vi "Optical Intrinsic Imaging with Optogenetic Stimulation_LED_3.0_w_Neuro.vi"() -> ()   [LabVIEW 2015]
uses:
  <vilib>/userdefined/High Color/IMAQdx.ctl
  <vilib>/vision/driver/IMAQdx.llb/IMAQdx Camera Control Mode.ctl
  <vilib>/DAQmx/write.llb/DAQmx Write (Analog 1D DBL 1Chan NSamp).vi
  <vilib>/DAQmx/read.llb/DAQmx Read (Analog 1D Wfm NChan NSamp).vi
  <vilib>/DAQmx/write.llb/DAQmx Write (Digital 1D Bool 1Chan 1Samp).vi
  <vilib>/DAQmx/create/channels.llb/DAQmx Create Channel (CO-Pulse Generation-Frequency).vi
  <vilib>/DAQmx/configure/timing.llb/DAQmx Timing (Implicit).vi
  <vilib>/DAQmx/create/channels.llb/DAQmx Create Channel (DO-Digital Output).vi
  <vilib>/DAQmx/create/channels.llb/DAQmx Create Channel (AI-Voltage-Basic).vi
  <vilib>/DAQmx/configure/timing.llb/DAQmx Timing (Sample Clock).vi
  <vilib>/DAQmx/configure/trigger.llb/DAQmx Start Trigger (Digital Edge).vi
  <vilib>/Waveform/DWDTOps.llb/DWDT Digital to Boolean Array.vi
  <vilib>/DAQmx/create/channels.llb/DAQmx Create Channel (AO-Voltage-Basic).vi
  <vilib>/DAQmx/miscellaneous.llb/DAQmx Fill In Error Info.vi
  <vilib>/vision/driver/NI_Vision_Acquisition_Software.lvlib
  <resource>/objmgr/daqmx.rc
panel:
  out "LED":bool
  out "Ball Velocity":waveform(dbl)(graph)={"t0"=timestamp(3636461995.1352177 s since 1904-01-01), "dt"=4.999999999999997e-05, "Y"=[-0.0010089086442716115, -0.001653132464493098, -0.0008478526887906051, -0.0008478526887906051, -0.001492076509693054, -0.001492076509693054, -0.0011699645995823372, -0.0008478526887906051, -0.0011699645995823372, -0.001492076509693054, -0.0013310205547228094], "attributes"=variant("NI_ChannelName"=variant(string "Dev1/ai0"), "NI_UnitDescription"=variant(string "Volts"))}
  out "Right Pad":bool
  out "Control":bool
  out "Left Pad":bool
  in  "Sol Stim Parameters":cluster{"Fs":dbl, "Samples":dbl}
  in  "LED Stim Parameters":cluster{"Fs":dbl, "Samples":dbl}
  in  "Sol Duty Cycle (%)":dbl=50.0
  in  "Sol Frequency":dbl=1.0
  in  "Sol Stim Duration (s)":dbl=1.0
  in  "LED duty cycle (%)":dbl=10.0
  in  "LED Frequency":dbl=10.0
  in  "LED Stim Duration (s)":dbl=2.0
  out "Stimulus Presentation Order":digitalwaveform[](graph)=[{"t0"=timestamp(0 s since 1904-01-01), "dt"=5e-05, "Y"={"transitions"=[], "data"=array6000000x1[6000000 elements]}}, {"t0"=timestamp(0 s since 1904-01-01), "dt"=5e-05, "Y"={"transitions"=[], "data"=array6000000x1[6000000 elements]}}, {"t0"=timestamp(0 s since 1904-01-01), "dt"=5e-05, "Y"={"transitions"=[], "data"=array6000000x1[6000000 elements]}}, {"t0"=timestamp(0 s since 1904-01-01), "dt"=5e-05, "Y"={"transitions"=[], "data"=array6000000x1[6000000 elements]}}]
  out "Solenoid Stim":digitalwaveform(graph)={"t0"=timestamp(0 s since 1904-01-01), "dt"=5e-05, "Y"={"transitions"=[], "data"=array20000x1[20000 elements]}}
  out "Dalsa Image":T1(plugin-control)
  in  "Trigger Solenoids":bool
  in  "WebCam\nFrame Rate":u32=15
  in  "Session Notes:":string[](array[string])=["QZ", "QZ_CHR01", "RH", "10", "0", "1", "n"]
  in  "Ai7":string="LED"
  in  "Ai6":string="MUA"
  in  "Ai5":string="LFP"
  in  "Ai4":string="Neuro\nSol"
  in  "Ai3":string="Right \nPad"
  in  "Ai2":string="Ctrl\nPad"
  in  "Ai1":string="Left Pad"
  in  "Ai0":string="VBall"
  in  "Flash LED":bool=TRUE
  in  "Trial Offset (s)":dbl=10.0
  in  "Time Between Stims (s)":dbl=30.0
  in  "Right Pad":dbl
  in  "Left Pad":dbl
  in  "Control":dbl
  in  "LED":dbl=5.0
  in  "Target Path":path=path "E:/Qingguang" caption="Final Saved Location for Files"
  in  "Analog Sampling Rate":dbl=20000.0 format="%0.0f"
  out "Analog file name":string="190326_12_18_1026"
  in  "physical channels":tag="Dev1/ai0:7"
  out "Actual WebCam Frame Rate":dbl(knob) scale=0.0..30.0
  out "WebCam":T1(plugin-control)
  out "Finished Acquiring":bool
  out "Trial Time Elapsed (Min)":cluster{dbl, dbl}(slide)={5.0, 1.6085833333333333} scale=0.0..5.0
  in  "Recording Time (min)":dbl=5.0 min=0.5 max=10.0 step=0.5
  in  "Temp Path":path=path "C:/LabView Direct Files" caption="Temporary Path for Streamed Data"
  in  "Dalsa\nFrame Rate":dbl=30.0
  out "Last Dalsa Buffer":i32=284
  in  "Stop":bool
  out "Actual Dalsa Frame Rate":dbl(knob) scale=0.0..60.0
  # "Experimenter"
  # "Animal ID"
  # "Imaged Hemisphere (RH/LH)"
  # "Solenoid Pressure (psi)"
  # "Isoflurane Time (military)"
  # "Session Number"
  # "Flash LEDs? (y/n)"
  # "Setup Stimulation:"
  # "File Settings:"
  # "Analog Acquisition Setup:"
  # "Camera Acquisition Setup:"
  # "BNC Pinout"
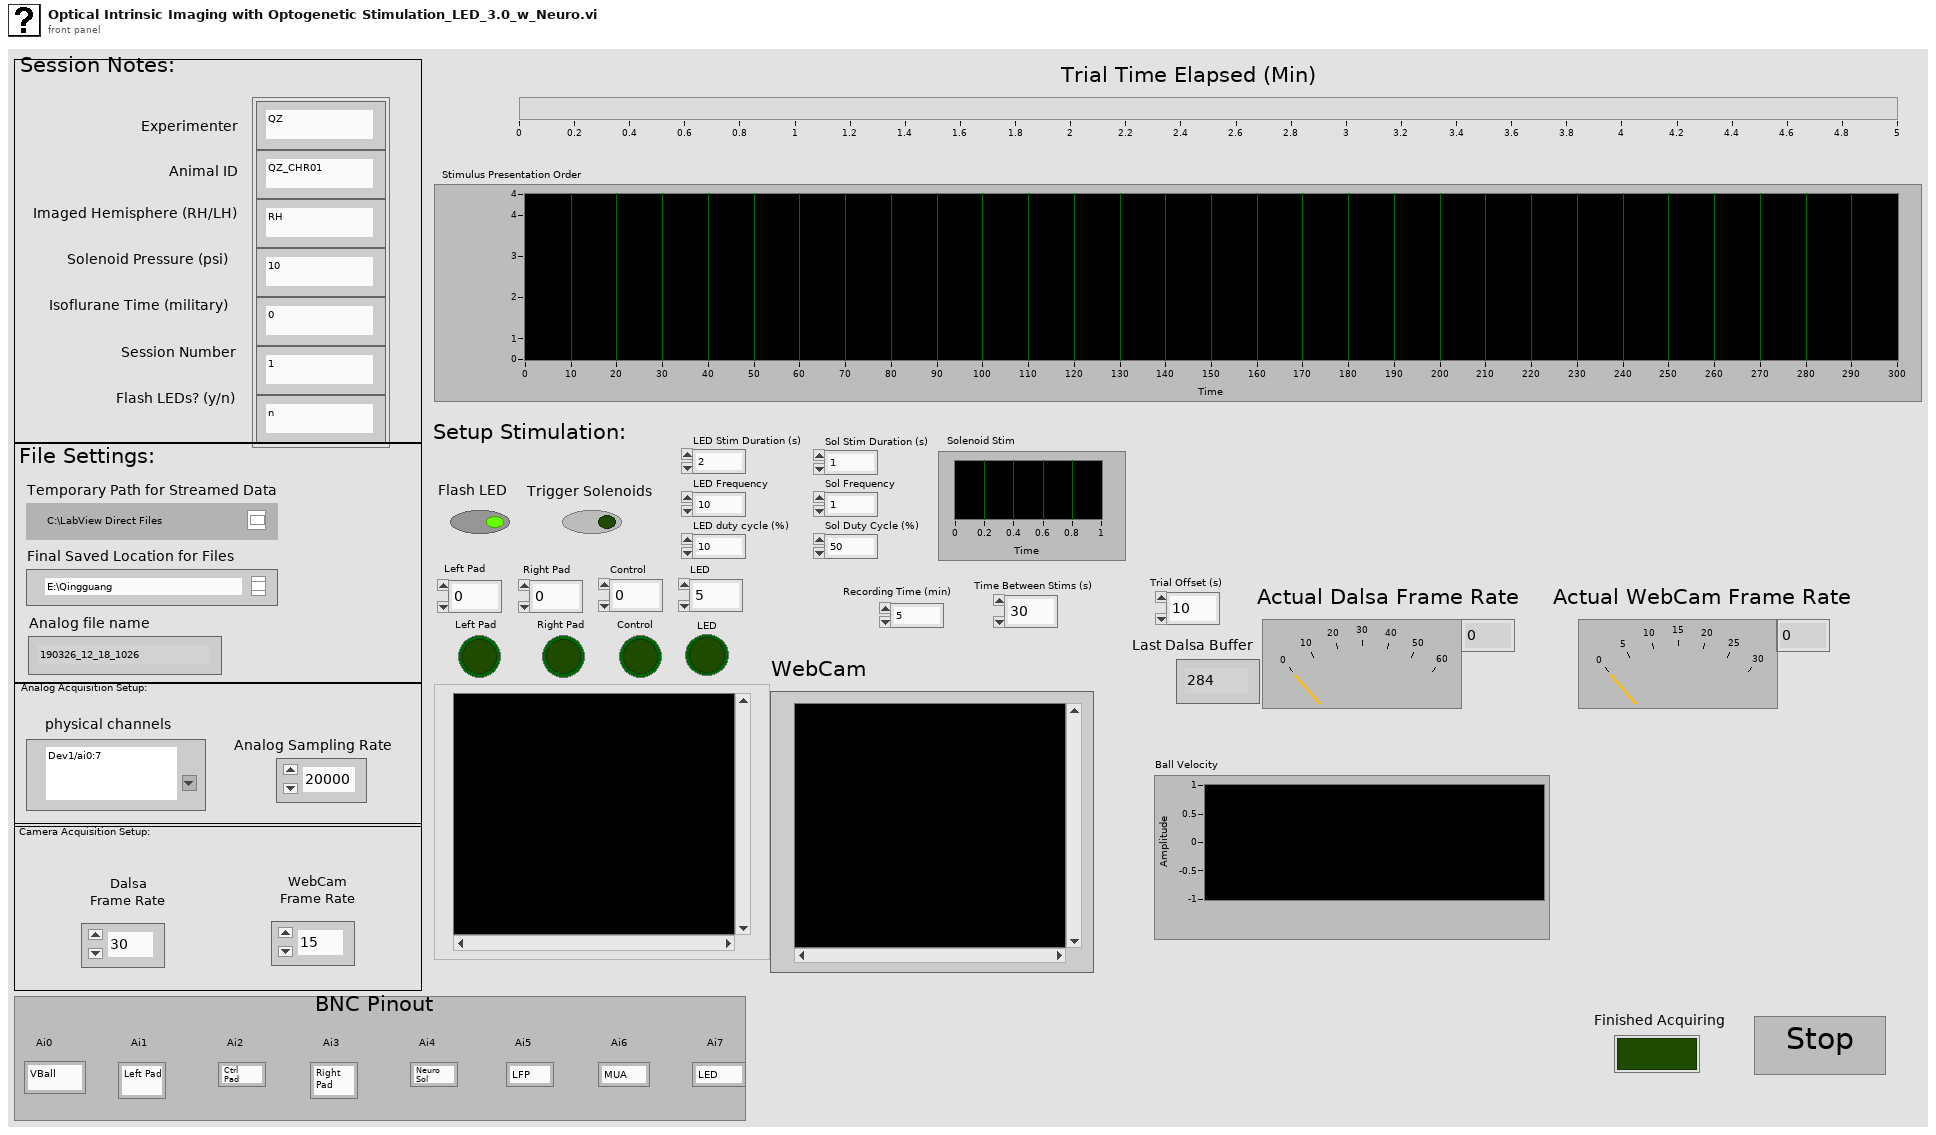
[diagram p1: front panel]
types:
  T1 = typedef "IMAQ Image.ctl" = refnum<image>
  T2 = typedef "Image Type" = u32
  T3 = typedef "NI_Vision_Acquisition_Software.lvlib/IMAQdx Camera Control Mode.ctl" = enum32{"Controller", "Listener"}
  T4 = typedef "IMAQdx.ctl" = refnum<k21>
  T5 = enum16{"open", "replace", "create", "open or create", "replace or create", "replace or create with confirmation"}
  T6 = typedef "AviRefnum.ctl" = refnum<k1>
  T7 = enum16{"big-endian, network order", "native, host order", "little-endian"}
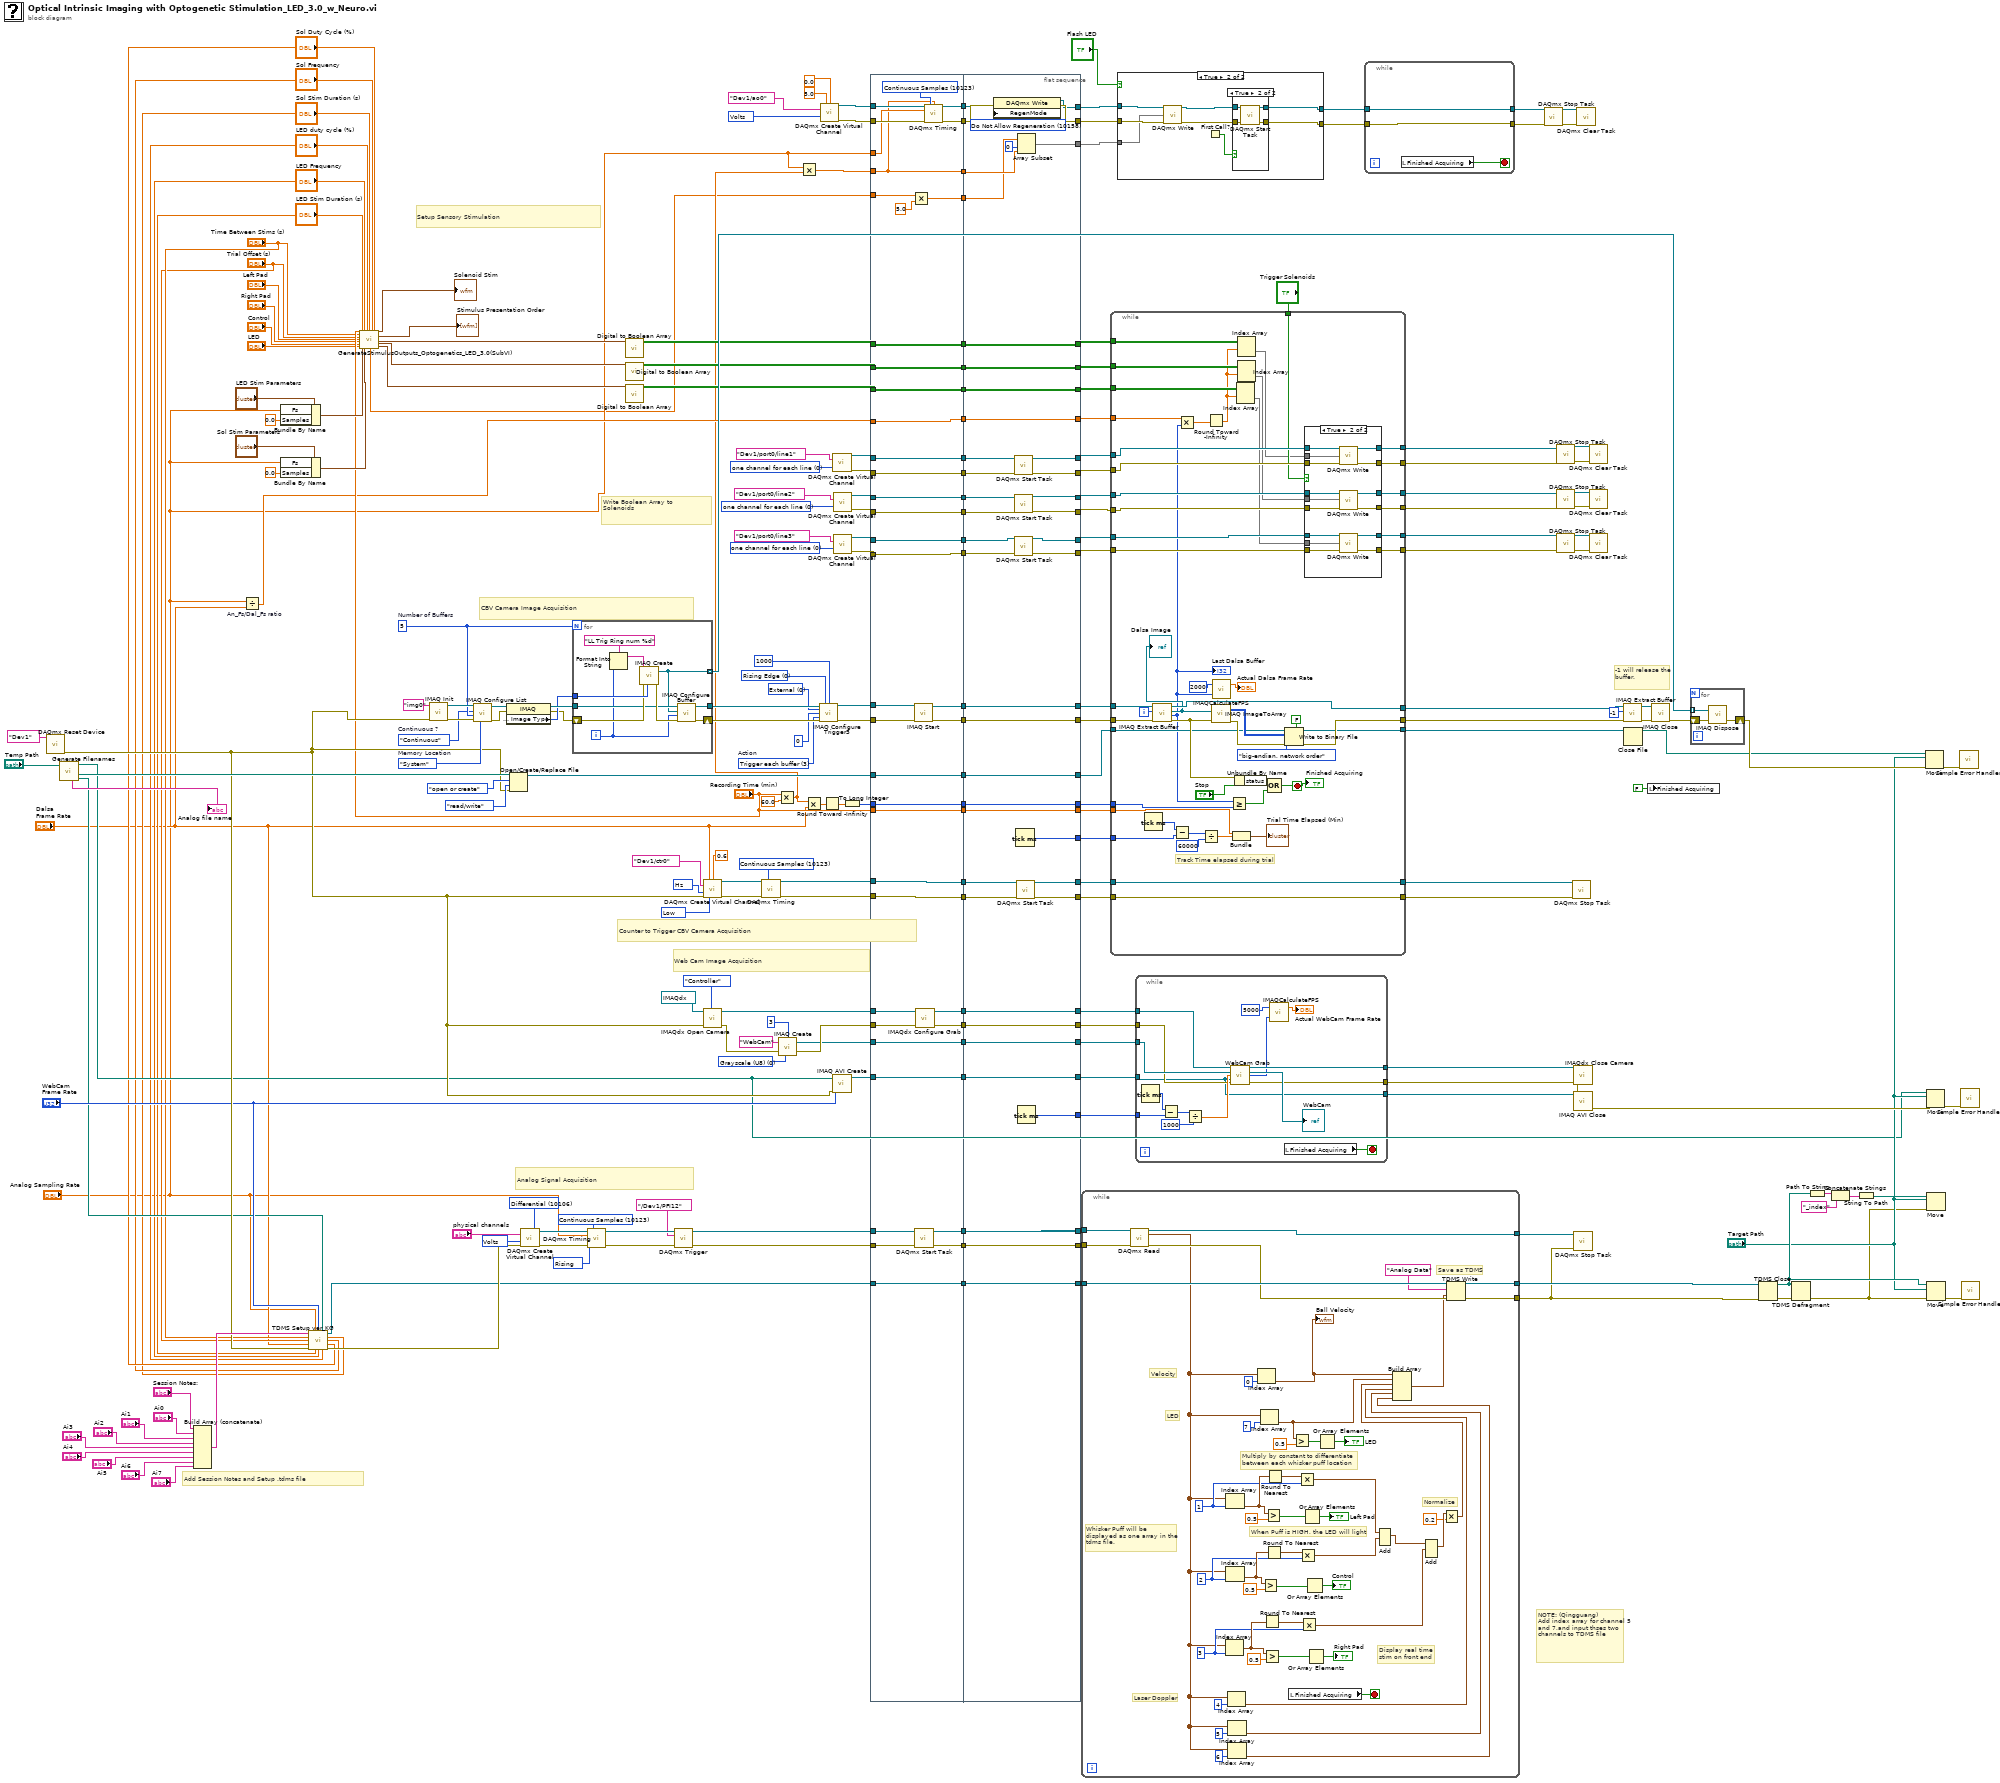
[diagram p0: block diagram]
diagram:
  w20 = 10348 items=["Volts"=10348, "From Custom Scale"=10065] ("units")
  w103 = 0 items=["one channel for each line", "one channel for all lines"] ("line grouping")
  w104 = 0 items=["one channel for each line", "one channel for all lines"] ("line grouping")
  w105 = 0 items=["one channel for each line", "one channel for all lines"] ("line grouping")
  w107 = 10348 items=["Volts"=10348, "From Custom Scale"=10065] ("units")
  w108 = 10280 items=["Rising"=10280, "Falling"=10171] ("active edge")
  w152 = 10123 items=["Finite Samples"=10178, "Continuous Samples"=10123, "Hardware Timed Single Point"=12522] ("sample mode")
  w155 = 10106 items=["default"=-1, "RSE"=10083, "NRSE"=10078, "Differential"=10106, "Pseudodifferential"=12529] ("input terminal configuration")
  w194 = T2 0 items=["Grayscale (U8)", "Grayscale (I16)", "Grayscale (SGL)", "Complex (CSG)", "RGB (U32)", "HSL (U32)", "RGB (U64)", "Grayscale (U16)"] ("Image Type")
  w217 = u32 0 items=["Rising Edge", "Falling Edge"] ("Trigger Polarity")
  w220 = u32 0 items=["External"=0, "RTSI"=1, "ISO In"=2, "Scaled Encoder"=5] ("Trigger Type")
  w210 = 10123 items=["Finite Samples"=10178, "Continuous Samples"=10123, "Hardware Timed Single Point"=12522] ("sample mode")
  w214 = 10373 items=["Hz"=10373] ("units")
  w215 = 10214 items=["High"=10192, "Low"=10214] ("idle state")
  w226 = u32 5  # Number of Buffers
  w218 = u32 3 items=["Disabled", "Trigger start of acquisition", "Trigger start of each buffer list", "Trigger each buffer", "Trigger each line (linescan)", "Trigger end of acquisition"]  # Action
  w225 = enum16{"System", "Onboard"}."System"  # Memory Location
  w224 = enum16{"One-Shot", "Continuous"}."Continuous"  # Continuous ?
  # "NOTE: (Qingguang)\nAdd index array for channel 5 and 7,and input thses two channels to TDMS file"
  # "Setup Sensory Stimulation"
  # "CBV Camera Image Acquisition"
  # "Counter to Trigger CBV Camera Acquisition"
  # "Web Cam Image Acquisition"
  # "Add Session Notes and Setup .tdms file"
  # "Analog Signal Acquisition"
  # "Write Boolean Array to \nSolenoids"
  # "-1 will release the buffer."
  n1 = call <vilib>:"DAQmx Reset Device.vi"("device in"=tag "Dev1") -> ("error out"=w53:errorcluster)  [unwired: 14 in]
  n2 = call "Generate Filenames.vi"("path"="Temp Path") -> ("TDMS Path"=w50:path, "Dalsa Path"=w202:path, "WebCam Path"=w49:path, "Analog file name"=→"Analog file name":string)  [unwired: 5 in, 2 out]
  n3 = Build Array (concatenate)("Session Notes:", "Ai0", "Ai1", "Ai2", "Ai3", "Ai4", "Ai5", "Ai6", "Ai7") -> (w55:string[])
  n4 = Divide "An_Fs/Dal_Fs ratio"(x="Analog Sampling Rate", y="Dalsa\nFrame Rate") -> (x/y=w26:dbl)
  n5 = Bundle By Name(cluster="LED Stim Parameters", "Fs"="Analog Sampling Rate", "Samples"=0.0) -> (w36:cluster{"Fs":dbl, "Samples":dbl})
  n6 = Bundle By Name(cluster="Sol Stim Parameters", "Fs"="Analog Sampling Rate", "Samples"=0.0) -> (w37:cluster{"Fs":dbl, "Samples":dbl})
  n7 = call "TDMS Setup ver_KG.vi"("Trial Notes"=w55, "Analog Sampling Rate"="Analog Sampling Rate", "WebCam Frame Rate"="WebCam\nFrame Rate", "file path"=w50, "Time between Stims"="Time Between Stims (s)", "Solenoid Duration"="Sol Stim Duration (s)", "Stim Offset"="Trial Offset (s)", "Solenoid Frequency"="Sol Frequency", "Dalsa Frame Rate"="Dalsa\nFrame Rate", "Solenoid Duty Cycle"="Sol Duty Cycle (%)", "error in (no error)"=w53, "LED Duration"="LED Stim Duration (s)", "LED Frequency"="LED Frequency", "LED Duty Cycle"="LED duty cycle (%)") -> ("tdms file out"=w51:refnum<k34>, "error out"=w54:errorcluster)
  n8 = call "GenerateStimulusOutputs_Optogenetics_LED_3.0(SubVI).vi"("Trial duration (min)"="Recording Time (min)", "Rest duration(s)"="Time Between Stims (s)", "trial offset (s)"="Trial Offset (s)", "Left Pad"="Left Pad", "Right Pad"="Right Pad", "Control"="Control", "LED"="LED", "LED Stim Duration (s)"="LED Stim Duration (s)", "LED Stim Parameters"=w36, "LED Frequency"="LED Frequency", "Sol Stim Parameters"=w37, "LED duty cycle (%)"="LED duty cycle (%)", "Sol Stim Duration (s)"="Sol Stim Duration (s)", "Sol Frequency"="Sol Frequency", "Sol Duty Cycle (%)"="Sol Duty Cycle (%)") -> ("Double LED Out"=w7:dbl[], "Solenoid Stim Waveforms"=→"Solenoid Stim":digitalwaveform, "Stimulus Digital Outputs"=→"Stimulus Presentation Order":digitalwaveform[], "Left Pad Out"=w48:digitalwaveform, "Control Out"=w47:digitalwaveform, "Right Pad Out"=w46:digitalwaveform)  [unwired: 5 in, 2 out]
  n9 = call <vilib>:"IMAQ Init.vi"("error in (no error)"=w53, "Interface Name"="img0") -> ("error out"=w236:errorcluster, "IMAQ Session Out"=w237:refnum<k11>)  [unwired: 8 out]
  n10 = call <vilib>:"IMAQ Configure List.vi"("Memory Location"=w225, "error in (no error)"=w236, "Number of buffers"=w226, "Continuous?"=w224, "IMAQ Session In"=w237) -> ("error out"=w234:errorcluster, "IMAQ Session Out"=w233:refnum<k11>)  [unwired: 1 in, 4 out]
  n11 = property class="IMAQ"(reference=w233, error in=w234) -> (reference out=w229:refnum<k11>, error out=w227:errorcluster, "Image Parameters : Image Type"=w228:u32)
  n12 = Open/Create/Replace File(file path (use dialog)=w202, error in=w53, operation (0:open)=T5."open or create", access (0:read/write)=enum16{"read/write", "read-only", "write-only"}."read/write") -> (refnum out=w156:refnum<file>)  [unwired: 2 in, 2 out]
  n13 = call-poly <vilib>:"DAQmx Create Virtual Channel.vi"("input terminal configuration"=w155, "physical channels"="physical channels", "units"=w107, "error in"=w54) -> ("task out"=w154:refnum<k21>, "error out"=w153:errorcluster)  [unwired: 10 in]
  n14 = for {
    N: w226 -> [_]
    tunnel: [w247] -> w222
    tunnel: w228 -> [w245]
    tunnel: w229 -> [w242]
    shift-right: [w246] -> w221
    shift-left: w227 -> [w244]
    tunnel: [w238] -> w223 mode=indexing
    i -> [w239]
    n15 = Format Into String(format string="LL Trig Ring num %d", w239) -> (resulting string=w241:string)  [unwired: 2 in, 1 out]
    n16 = call "IMAQ Create"("Image Name"=w241, "Image Type"=w245, "error in (no error)"=w244) -> ("New Image"=w238:T1, "error out"=w243:errorcluster)  [unwired: 1 in, 1 out]
    n17 = call <vilib>:"IMAQ Configure Buffer.vi"("error in (no error)"=w243, "Buffer Number"=w239, "Image In"=w238, "IMAQ Session In"=w242) -> ("error out"=w246:errorcluster, "IMAQ Session Out"=w247:refnum<k11>)  [unwired: 2 in, 4 out]
  }
  n18 = call-poly <vilib>:"DAQmx Timing.vi"("task/channels in"=w154, "sample mode"=w152, "rate"="Analog Sampling Rate", "active edge"=w108, "error in"=w153) -> ("task out"=w151:refnum<k21>, "error out"=w150:errorcluster)  [unwired: 9 in]
  n19 = call-poly <vilib>:"Digital to Boolean Array.vi"("digital waveform"=w48) -> ("boolean array"=w66:bool[][])  [unwired: 9 in, 1 out]
  n20 = call-poly <vilib>:"Digital to Boolean Array.vi"("digital waveform"=w47) -> ("boolean array"=w63:bool[][])  [unwired: 9 in, 1 out]
  n21 = call-poly <vilib>:"Digital to Boolean Array.vi"("digital waveform"=w46) -> ("boolean array"=w61:bool[][])  [unwired: 9 in, 1 out]
  n22 = call-poly <vilib>:"DAQmx Trigger.vi"("task/channels in"=w151, "source"=tag "/Dev1/PFI12", "error in"=w150) -> ("task out"=w148:refnum<k21>, "error out"=w147:errorcluster)  [unwired: 11 in]
  n23 = call-poly <vilib>:"DAQmx Create Virtual Channel.vi"("frequency"="Dalsa\nFrame Rate", "duty cycle"=0.6, "counter"=tag "Dev1/ctr0", "units"=w214, "error in"=w53, "idle state"=w215) -> ("task out"=w212:refnum<k21>, "error out"=w211:errorcluster)  [unwired: 8 in]
  n24 = call <vilib>:"IMAQdx Open Camera.vi"("Camera Control Mode"=IMAQdx_Camera_Control_Mode."Controller", "error in"=w53, "Session In"=T4 "cam0") -> ("error out"=w190:errorcluster, "Session Out"=w188:T4)  [unwired: 7 in]
  n25 = call-poly <vilib>:"DAQmx Timing.vi"("task/channels in"=w212, "sample mode"=w210, "error in"=w211) -> ("task out"=w138:refnum<k21>, "error out"=w136:errorcluster)  [unwired: 11 in]
  n26 = Multiply(x="Recording Time (min)", y=60.0) -> (x*y=w16:dbl)
  n27 = call "IMAQ Create"("Border Size"=3, "Image Name"="WebCam", "Image Type"=w194, "error in (no error)"=w190) -> ("New Image"=w187:T1, "error out"=w189:errorcluster)  [unwired: 1 in]
  n28 = Multiply(x="Analog Sampling Rate", y=w16) -> (x*y=w14:dbl)
  n29 = Multiply(x=w16, y="Dalsa\nFrame Rate") -> (x*y=w199:dbl)
  n30 = call <vilib>:"IMAQ Configure Trigger3.vi"("IMAQ Session In"=w222, "Polarity"=w217, "Frame timeout (ms)"=u32 1000 ("Frame Timeout (ms)"), "Type"=w220, "Line Number"=u32 0 ("Trigger Line Number"), "Action"=w218, "error in (no error)"=w221) -> ("IMAQ Session Out"=w174:refnum<k11>, "error out"=w173:errorcluster)  [unwired: 2 in, 5 out]
  n31 = call-poly <vilib>:"DAQmx Create Virtual Channel.vi"("maximum value"=5.0, "minimum value"=0.0, "physical channels"=tag "Dev1/ao0", "units"=w20) -> ("task out"=w17:refnum<k21>, "error out"=w18:errorcluster)  [unwired: 10 in]
  n32 = Round Toward -Infinity(1:w199) -> (0:w198:dbl)
  n33 = call-poly <vilib>:"DAQmx Create Virtual Channel.vi"("lines"=tag "Dev1/port0/line1", "line grouping"=w103) -> ("task out"=w98:refnum<k21>, "error out"=w95:errorcluster)  [unwired: 12 in]
  n34 = call "IMAQ AVI Create"("error in (no error)"=w53, "Frames Per Second"="WebCam\nFrame Rate", "AVI Path"=w49) -> ("Avi Refnum"=w180:T6)  [unwired: 7 in, 1 out]
  n35 = call-poly <vilib>:"DAQmx Create Virtual Channel.vi"("lines"=tag "Dev1/port0/line2", "line grouping"=w104) -> ("task out"=w92:refnum<k21>, "error out"=w90:errorcluster)  [unwired: 12 in]
  n36 = call-poly <vilib>:"DAQmx Create Virtual Channel.vi"("lines"=tag "Dev1/port0/line3", "line grouping"=w105) -> ("task out"=w86:refnum<k21>, "error out"=w83:errorcluster)  [unwired: 12 in]
  n37 = To Long Integer(number=w198) -> (32bit integer=w163:i32)
  n38 = flat-sequence {
    tunnel: w189 -> [w287]
    tunnel: w188 -> [w286]
    tunnel: w187 -> [w285]
    tunnel: [w285] -> w186
    tunnel: [w284] -> w184
    tunnel: [w283] -> w182
    tunnel: w180 -> [w282]
    tunnel: [w282] -> w179
    tunnel: w174 -> [w281]
    tunnel: w173 -> [w280]
    tunnel: [w279] -> w171
    tunnel: [w278] -> w169
    tunnel: w163 -> [w277]
    tunnel: [w277] -> w162
    tunnel: "Recording Time (min)" -> [w276]
    tunnel: [w276] -> w159
    tunnel: [w275] -> w157
    tunnel: w156 -> [w275]
    tunnel: w148 -> [w274]
    tunnel: w147 -> [w273]
    tunnel: [w272] -> w146
    tunnel: [w271] -> w145
    tunnel: [w270] -> w140
    tunnel: w51 -> [w270]
    tunnel: w138 -> [w269]
    tunnel: [w269] -> w137
    tunnel: w136 -> [w268]
    tunnel: [w268] -> w135
    tunnel: [w267] -> w99
    tunnel: w98 -> [w267]
    tunnel: [w266] -> w96
    tunnel: w95 -> [w266]
    tunnel: [w265] -> w93
    tunnel: w92 -> [w265]
    tunnel: w90 -> [w264]
    tunnel: [w264] -> w89
    tunnel: [w263] -> w87
    tunnel: w86 -> [w263]
    tunnel: [w262] -> w84
    tunnel: w83 -> [w262]
    tunnel: [w261] -> w67
    tunnel: w66 -> [w261]
    tunnel: [w260] -> w64
    tunnel: w63 -> [w260]
    tunnel: w61 -> [w259]
    tunnel: [w259] -> w60
    tunnel: [w258] -> w27
    tunnel: w26 -> [w258]
    tunnel: w18 -> [w256]
    tunnel: w17 -> [w255]
    tunnel: "Analog Sampling Rate" -> [w254]
    tunnel: w14 -> [w251]
    tunnel: [w253] -> _
    tunnel: [w253] -> w13
    tunnel: [w252] -> w12
    tunnel: [w251] -> w9
    tunnel: w7 -> [w249]
    tunnel: [w248] -> w6
    tunnel: [w330] -> w191
    tunnel: w186 -> [w329]
    tunnel: [w329] -> w185
    tunnel: w184 -> [w328]
    tunnel: [w328] -> w183
    tunnel: w182 -> [w327]
    tunnel: [w327] -> w181
    tunnel: w179 -> [w326]
    tunnel: [w326] -> w178
    tunnel: [w325] -> w172
    tunnel: w171 -> [w325]
    tunnel: [w324] -> w170
    tunnel: w169 -> [w324]
    tunnel: [w316] -> w167
    tunnel: [w315] -> w165
    tunnel: [w323] -> w164
    tunnel: w162 -> [w322]
    tunnel: [w322] -> w161
    tunnel: [w321] -> w160
    tunnel: w159 -> [w321]
    tunnel: [w320] -> w158
    tunnel: w157 -> [w320]
    tunnel: [w319] -> w143
    tunnel: w146 -> [w319]
    tunnel: [w318] -> w144
    tunnel: w145 -> [w318]
    tunnel: [w317] -> w141
    tunnel: w140 -> [w317]
    tunnel: w137 -> [w314]
    tunnel: w135 -> [w313]
    tunnel: w99 -> [w311]
    tunnel: [w310] -> w97
    tunnel: w96 -> [w309]
    tunnel: [w308] -> w94
    tunnel: w93 -> [w307]
    tunnel: [w306] -> w91
    tunnel: w89 -> [w305]
    tunnel: [w304] -> w88
    tunnel: w87 -> [w303]
    tunnel: [w312] -> w85
    tunnel: w84 -> [w302]
    tunnel: [w301] -> w82
    tunnel: w67 -> [w300]
    tunnel: [w300] -> w65
    tunnel: w64 -> [w299]
    tunnel: [w299] -> w62
    tunnel: [w298] -> w59
    tunnel: w60 -> [w298]
    tunnel: w27 -> [w297]
    tunnel: [w297] -> w25
    tunnel: w13 -> [w289]
    tunnel: [w288] -> w11
    tunnel: w12 -> [w291]
    tunnel: [w290] -> w10
    tunnel: w9 -> [w295]
    tunnel: [w294] -> w8
    tunnel: w6 -> [w293]
    frame #0 {
      w257 = 10123 items=["Finite Samples"=10178, "Continuous Samples"=10123, "Hardware Timed Single Point"=12522] ("sample mode")
      n39 = Multiply(x=w249, y=5.0) -> (x*y=w248:dbl[])
      n40 = call <vilib>:"IMAQ Start.vi"("error in (no error)"=w280, "IMAQ Session In"=w281) -> ("error out"=w278:errorcluster, "IMAQ Session Out"=w279:refnum<k11>)  [unwired: 8 out]
      n41 = call <vilib>:"DAQmx Start Task.vi"("task/channels in"=w274, "error in"=w273) -> ("task out"=w272:refnum<k21>, "error out"=w271:errorcluster)  [unwired: 12 in]
      n42 = call <vilib>:"IMAQdx Configure Grab.vi"("error in"=w287, "Session In"=w286) -> ("error out"=w283:errorcluster, "Session Out"=w284:T4)  [unwired: 8 in]
      n43 = call-poly <vilib>:"DAQmx Timing.vi"("task/channels in"=w255, "sample mode"=w257, "samples per channel"=w251, "rate"=w254, "error in"=w256) -> ("task out"=w253:refnum<k21>, "error out"=w252:errorcluster)  [unwired: 9 in]
    }
    frame #1 {
      w292 = 10158 items=["Allow Regeneration"=10097, "Do Not Allow Regeneration"=10158] ("RegenMode")
      n44 = property class="DAQmx Write"(reference=w289, error in=w291, "RegenMode"=w292) -> (reference out=w288:refnum<k21>, error out=w290:errorcluster)
      n45 = call <vilib>:"DAQmx Start Task.vi"("task/channels in"=w311, "error in"=w309) -> ("task out"=w310:refnum<k21>, "error out"=w308:errorcluster)  [unwired: 12 in]
      n46 = call <vilib>:"DAQmx Start Task.vi"("task/channels in"=w307, "error in"=w305) -> ("task out"=w306:refnum<k21>, "error out"=w304:errorcluster)  [unwired: 12 in]
      n47 = call <vilib>:"DAQmx Start Task.vi"("task/channels in"=w303, "error in"=w302) -> ("task out"=w312:refnum<k21>, "error out"=w301:errorcluster)  [unwired: 12 in]
      n48 = Tick Count (ms)() -> (millisecond timer value=w323:u32)
      n49 = call <vilib>:"DAQmx Start Task.vi"("task/channels in"=w314, "error in"=w313) -> ("task out"=w316:refnum<k21>, "error out"=w315:errorcluster)  [unwired: 12 in]
      n50 = Array Subset(array=w293, index=0, length=w295) -> (w294:dbl[])
      n51 = Tick Count (ms)() -> (millisecond timer value=w330:u32)
    }
  }
  n52 = while {
    tunnel: w144 -> [w379]
    tunnel: w143 -> [w378]
    tunnel: w141 -> [w377]
    tunnel: [w376] -> w110
    tunnel: [w375] -> w109
    tunnel: [w374] -> w139
    stop <- w373 stop-if-true
    w354 = 3 ("index")
    w356 = 2 ("index")
    w359 = 1 ("index")
    # "Laser Doppler"
    # "Save as TDMS"
    # "LED"
    # "Velocity"
    # "When Puff is HIGH, the LED will light"
    # "Normalize"
    # "Multiply by constant to differentiate \nbetween each whisker puff location"
    # "Whisker Puff will be\ndisplayed as one array in the\ntdms file."
    # "Display real time\nstim on front end"
    n53 = call-poly <vilib>:"DAQmx Read.vi"("task/channels in"=w378, "error in"=w379) -> ("task out"=w374:refnum<k21>, "data"=w335:waveform(dbl)[], "error out"=w371:errorcluster)  [unwired: 11 in]
    n54 = Index Array(array=w335, index=w354) -> (element=w355:waveform(dbl))
    n55 = Index Array(array=w335, index=w359) -> (element=w361:waveform(dbl))
    n56 = Index Array(array=w335, index=w356) -> (element=w358:waveform(dbl))
    n57 = Index Array(array=w335, index=4) -> (element=w336:waveform(dbl))
    n58 = Index Array(array=w335, index=5) -> (element=w332:waveform(dbl))
    n59 = Index Array(array=w335, index=6) -> (element=w331:waveform(dbl))
    n60 = Index Array(array=w335, index=0) -> (element=w344:waveform(dbl))
    "Ball Velocity" <- w344
    n61 = Index Array(array=w335, index=7) -> (element=w341:waveform(dbl))
    n62 = Greater?(x=w358, y=0.5) -> (0:w365:bool[])
    n63 = Round To Nearest(number=w355) -> (nearest integer value=w353:waveform(dbl))
    n64 = Greater?(x=w355, y=0.5) -> (0:w363:bool[])
    n65 = Greater?(x=w361, y=0.5) -> (0:w369:bool[])
    n66 = Round To Nearest(number=w358) -> (nearest integer value=w357:waveform(dbl))
    n67 = Round To Nearest(number=w361) -> (nearest integer value=w360:waveform(dbl))
    n68 = local read "Finished Acquiring"() -> (w373:bool)
    n69 = Greater?(x=w341, y=0.5) -> (0:w340:bool[])
    n70 = Multiply(x=w360, y=w359) -> (x*y=w352:waveform(dbl))
    n71 = Multiply(x=w357, y=w356) -> (x*y=w351:waveform(dbl))
    n72 = Multiply(x=w353, y=w354) -> (x*y=w350:waveform(dbl))
    n73 = Or Array Elements(Boolean array=w369) -> (logical OR=→"Left Pad":bool)
    n74 = Or Array Elements(Boolean array=w365) -> (logical OR=→"Control":bool)
    n75 = Or Array Elements(Boolean array=w363) -> (logical OR=→"Right Pad":bool)
    n76 = Or Array Elements(Boolean array=w340) -> (logical OR=→"LED":bool)
    n77 = Add(1:w351, 2:w352) -> (0:w349:waveform(dbl))  [unwired: 1 in, 1 out]
    n78 = Add(1:w350, 2:w349) -> (0:w348:waveform(dbl))  [unwired: 1 in, 1 out]
    n79 = Multiply(x=w348, y=0.2) -> (x*y=w346:waveform(dbl))
    n80 = Build Array(w344, w341, w346, w336, w332, w331) -> (w338:waveform(dbl)[])
    n81 = TDMS Write(0:w377, 5:"Analog Data" ("group name in (Untitled)"), 9:w338, 11:w371) -> (4:w376:refnum<k34>, 15:w375:errorcluster)  [unwired: 2 in, 2 out]
  }
  n82 = while {
    tunnel: w172 -> [w430]
    tunnel: w170 -> [w431]
    tunnel: [w425] -> w204
    tunnel: [w423] -> w205
    tunnel: [w422] -> w203
    tunnel: [w413] -> w168
    tunnel: w167 -> [w413]
    tunnel: [w412] -> w166
    tunnel: w165 -> [w412]
    tunnel: w164 -> [w411]
    tunnel: w161 -> [w410]
    tunnel: w160 -> [w409]
    tunnel: w158 -> [w407]
    tunnel: w97 -> [w394]
    tunnel: w94 -> [w393]
    tunnel: w91 -> [w398]
    tunnel: w88 -> [w397]
    tunnel: w85 -> [w402]
    tunnel: w82 -> [w401]
    tunnel: [w400] -> w81
    tunnel: [w399] -> w80
    tunnel: [w396] -> w79
    tunnel: [w395] -> w78
    tunnel: [w392] -> w77
    tunnel: [w391] -> w76
    tunnel: w65 -> [w385]
    tunnel: w62 -> [w387]
    tunnel: w59 -> [w389]
    tunnel: "Trigger Solenoids" -> [w390]
    tunnel: w25 -> [w382]
    i -> [w429]
    stop <- w414 stop-if-true
    # "Track Time elapsed during trial"
    n83 = Tick Count (ms)() -> (millisecond timer value=w419:u32)
    n84 = call <vilib>:"IMAQ Extract Buffer.vi"("error in (no error)"=w431, "Buffer to extract"=w429, "IMAQ Session In"=w430) -> ("error out"=w420:errorcluster, "Buffer Number"=w383:i32, "Image Out"=w403:T1, "IMAQ Session Out"=w423:refnum<k11>)  [unwired: 5 out]
    "Last Dalsa Buffer" <- w383
    "Dalsa Image" <- w403
    n85 = Subtract(x=w419, y=w411) -> (x-y=w418:u32)
    n86 = Multiply(x=w382, y=w383) -> (x*y=w381:dbl)
    n87 = Divide(x=w418, y=u32 60000) -> (x/y=w416:dbl)
    n88 = Round Toward -Infinity(1:w381) -> (0:w380:dbl)
    n89 = call "IMAQ ImageToArray"("error in (no error)"=w420, "Image"=w403) -> ("error out"=w428:errorcluster, "Image Pixels (I16)"=w427:i16[][])  [unwired: 2 in, 3 out]
    n90 = call "IMAQCalculateFPS.vi"("Update interval"=w383, "buffer number"=u32 2000 ("Update Interval (ms)")) -> ("acquired FPS"=→"Actual Dalsa Frame Rate":dbl)  [unwired: 1 out]
    n91 = Greater Or Equal?(x=w383, y=w410) -> (x >= y?=w415:bool)
    n92 = Bundle("Recording Time (min)"=w409, w416) -> (→"Trial Time Elapsed (Min)":cluster{"Recording Time (min)":dbl, dbl})  [unwired: 1 in]
    n93 = Unbundle By Name(w420) -> ("status"=w405:bool)
    n94 = Index Array(array=w389, index (row)=w380) -> (element=w388:bool[])  [unwired: 1 in]
    n95 = Index Array(array=w385, index (row)=w380) -> (element=w384:bool[])  [unwired: 1 in]
    n96 = Index Array(array=w387, index (row)=w380) -> (element=w386:bool[])  [unwired: 1 in]
    n97 = Compound Arithmetic op=OR(w405, "Stop", w415) -> (w414:bool)
    "Finished Acquiring" <- w414
    n98 = Write to Binary File(file (use dialog)=w407, data=w427, error in=w428, 5:FALSE ("prepend array or string size? (T)"), 9:T7."big-endian, network order" ("byte order (0:big-endian, network order)")) -> (refnum out=w422:refnum<file>, error out=w425:errorcluster)  [unwired: 1 in, 1 out]
    n99 = case shown="True" w390 {
      tunnel: w402 -> [w433 w452]
      tunnel: w401 -> [w432 w451]
      tunnel: [w433 w450] -> w400
      tunnel: [w432 w449] -> w399
      tunnel: w398 -> [w435 w448]
      tunnel: w397 -> [w434 w447]
      tunnel: [w435 w446] -> w396
      tunnel: [w434 w445] -> w395
      tunnel: w394 -> [w437 w444]
      tunnel: w393 -> [w436 w443]
      tunnel: [w437 w442] -> w392
      tunnel: [w436 w441] -> w391
      tunnel: w388 -> [_ w440]
      tunnel: w386 -> [_ w439]
      tunnel: w384 -> [_ w438]
      frame False {
      }
      frame True {
        n100 = call-poly <vilib>:"DAQmx Write.vi"("task/channels in"=w444, "data"=w438, "error in"=w443) -> ("task out"=w442:refnum<k21>, "error out"=w441:errorcluster)  [unwired: 10 in, 1 out]
        n101 = call-poly <vilib>:"DAQmx Write.vi"("task/channels in"=w448, "data"=w439, "error in"=w447) -> ("task out"=w446:refnum<k21>, "error out"=w445:errorcluster)  [unwired: 10 in, 1 out]
        n102 = call-poly <vilib>:"DAQmx Write.vi"("task/channels in"=w452, "data"=w440, "error in"=w451) -> ("task out"=w450:refnum<k21>, "error out"=w449:errorcluster)  [unwired: 10 in, 1 out]
      }
    }
  }
  n103 = case shown="True" "Flash LED" {
    tunnel: [w454 w461] -> w3
    tunnel: [w453 w460] -> w2
    tunnel: w11 -> [w454 w459]
    tunnel: w10 -> [w453 w458]
    tunnel: w8 -> [_ w457]
    frame False {
    }
    frame True {
      n104 = call-poly <vilib>:"DAQmx Write.vi"("task/channels in"=w459, "data"=w457, "error in"=w458) -> ("task out"=w455:refnum<k21>, "error out"=w462:errorcluster)  [unwired: 10 in, 1 out]
      n105 = First Call?() -> (First Call?: T/F=w456:bool)
      n106 = case shown="True" w456 {
        tunnel: w455 -> [w463 w468]
        tunnel: w462 -> [w464 w467]
        tunnel: [w463 w466] -> w461
        tunnel: [w464 w465] -> w460
        frame False {
        }
        frame True {
          n107 = call <vilib>:"DAQmx Start Task.vi"("task/channels in"=w468, "error in"=w467) -> ("task out"=w466:refnum<k21>, "error out"=w465:errorcluster)  [unwired: 12 in]
        }
      }
    }
  }
  n108 = while {
    tunnel: w191 -> [w479]
    tunnel: w185 -> [w477]
    tunnel: w183 -> [w476]
    tunnel: w181 -> [w475]
    tunnel: w178 -> [w470]
    tunnel: [w473] -> w177
    tunnel: [w472] -> w175
    tunnel: [w470] -> w176
    stop <- w481 stop-if-true
    n109 = Tick Count (ms)() -> (millisecond timer value=w482:u32)
    n110 = Subtract(x=w482, y=w479) -> (x-y=w483:u32)
    n111 = Divide(x=w483, y=u32 1000) -> (x/y=w478:dbl)
    n112 = call "WebCam Grab.vi"("Session In"=w476, "Image In"=w477, "Trial Time"=w478, "Avi Refnum"=w470, "error in"=w475) -> ("Session Out"=w473:T4, "WebCam Img Out"=→"WebCam":T1, "Buffer Number Out"=w471:u32, "error out"=w472:errorcluster)  [unwired: 7 in]
    n113 = call "IMAQCalculateFPS.vi"("Update interval"=w471, "buffer number"=u32 5000 ("Update Interval (ms)")) -> ("acquired FPS"=→"Actual WebCam Frame Rate":dbl)  [unwired: 1 out]
    n114 = local read "Finished Acquiring"() -> (w481:bool)
  }
  n115 = while {
    tunnel: [w487] -> w4
    tunnel: w3 -> [w487]
    tunnel: w2 -> [w486]
    tunnel: [w486] -> w1
    stop <- w485 stop-if-true
    n116 = local read "Finished Acquiring"() -> (w485:bool)
  }
  n117 = call <vilib>:"DAQmx Stop Task.vi"("task/channels in"=w4, "error in"=w1) -> ("task out"=w23:refnum<k21>, "error out"=w22:errorcluster)  [unwired: 12 in]
  n118 = call <vilib>:"DAQmx Stop Task.vi"("task/channels in"=w77, "error in"=w76) -> ("task out"=w71:refnum<k21>, "error out"=w70:errorcluster)  [unwired: 12 in]
  n119 = call <vilib>:"DAQmx Stop Task.vi"("task/channels in"=w79, "error in"=w78) -> ("task out"=w73:refnum<k21>, "error out"=w72:errorcluster)  [unwired: 12 in]
  n120 = call <vilib>:"DAQmx Stop Task.vi"("task/channels in"=w81, "error in"=w80) -> ("task out"=w75:refnum<k21>, "error out"=w74:errorcluster)  [unwired: 12 in]
  n121 = call <vilib>:"DAQmx Stop Task.vi"("task/channels in"=w168, "error in"=w166) -> ()  [unwired: 12 in, 2 out]
  n122 = call <vilib>:"IMAQdx Close Camera.vi"("error in"=w175, "Session In"=w177) -> ()  [unwired: 9 in, 1 out]
  n123 = call "IMAQ AVI Close"("error in (no error)"=w175, "Avi Refnum"=w176) -> ("error out"=w130:errorcluster)  [unwired: 9 in]
  n124 = call <vilib>:"DAQmx Stop Task.vi"("task/channels in"=w139, "error in"=w109) -> ()  [unwired: 12 in, 2 out]
  n125 = call <vilib>:"DAQmx Clear Task.vi"("task in"=w23, "error in"=w22) -> ()  [unwired: 13 in, 1 out]
  n126 = call <vilib>:"DAQmx Clear Task.vi"("task in"=w71, "error in"=w70) -> ()  [unwired: 13 in, 1 out]
  n127 = call <vilib>:"DAQmx Clear Task.vi"("task in"=w73, "error in"=w72) -> ()  [unwired: 13 in, 1 out]
  n128 = call <vilib>:"DAQmx Clear Task.vi"("task in"=w75, "error in"=w74) -> ()  [unwired: 13 in, 1 out]
  n129 = call <vilib>:"IMAQ Extract Buffer.vi"("error in (no error)"=w204, "Buffer to extract"=-1, "IMAQ Session In"=w205) -> ("error out"=w231:errorcluster, "IMAQ Session Out"=w230:refnum<k11>)  [unwired: 7 out]
  n130 = Close File(refnum=w203) -> (path=w131:path)  [unwired: 1 in, 1 out]
  n131 = local write "Finished Acquiring"(FALSE ("Finished Acquiring")) -> ()
  n132 = call <vilib>:"IMAQ Close.vi"("error in (no error)"=w231, "IMAQ Session In"=w230) -> ("error out"=w235:errorcluster)  [unwired: 9 out]
  n133 = for {
    tunnel: w223 -> [w490] mode=indexing
    shift-right: [w488] -> w133
    shift-left: w235 -> [w489]
    n134 = call "IMAQ Dispose"("Image"=w490, "error in (no error)"=w489) -> ("error out"=w488:errorcluster)  [unwired: 1 in, 3 out]
  }
  n135 = TDMS Close(8:w109, 11:w110) -> (0:w134:errorcluster, 3:w125:path)
  n136 = TDMS Defragment(4:w134, 7:w125) -> (0:w121:errorcluster)
  n137 = Path To String(path=w125) -> (string=w127:string)
  n138 = Concatenate Strings(w127, "_index" ("string")) -> (w124:string)
  n139 = String To Path(string=w124) -> (path=w123:path)
  n140 = Move(source path=w131, error in=w133, 10:"Target Path") -> (error out=w132:errorcluster)  [unwired: 2 in, 2 out]
  n141 = Move(source path=w49, error in=w130, 10:"Target Path") -> (error out=w128:errorcluster)  [unwired: 2 in, 2 out]
  n142 = Move(source path=w123, error in=w121, 10:"Target Path") -> ()  [unwired: 2 in, 3 out]
  n143 = Move(source path=w125, error in=w121, 10:"Target Path") -> (error out=w129:errorcluster)  [unwired: 2 in, 2 out]
  n144 = call <vilib>:"Simple Error Handler.vi"("error in (no error)"=w132) -> ()  [unwired: 1 in, 8 out]
  n145 = call <vilib>:"Simple Error Handler.vi"("error in (no error)"=w128) -> ()  [unwired: 1 in, 8 out]
  n146 = call <vilib>:"Simple Error Handler.vi"("error in (no error)"=w129) -> ()  [unwired: 1 in, 8 out]
